vi "linear interp iiii- complex - z-omega - tails.vi"(0 "z":cdb[](array[numeric]), 5 "omega":dbl[](array[numeric]), 11 "center":i32=-1) -> (2 "directed sigma":cdb, 3 "directed sigma - abs":dbl, 4 "z out":cdb[](array[numeric]), 6 "omega out":dbl[](array[numeric]), 8 "left":cdb, 10 "center":cdb, 12 "intercept":cdb, 13 "slope":cdb, 15 "right":cdb)   [LabVIEW 2010]
uses:
  Q - not nan -- real.vi
  Q - not nan -- integer.vi
  <vilib>/Analysis/Matrix/Numeric/Conversions/Array To Matrix - RA2.vi
  <vilib>/Analysis/baseanly.llb/Real Inverse Matrix.vi
  <vilib>/Analysis/7linalg.llb/Real Eigenvalues and Vectors.vi
  <vilib>/Analysis/Matrix/Numeric/Conversions/Matrix To Array - CM.vi
  <vilib>/Analysis/baseanly.llb/Complex A x B.vi
  <vilib>/Analysis/NI_AALBase.lvlib
  <vilib>/Analysis/Matrix/NI_Matrix.lvlib
  <vilib>/Analysis/NI_AALPro.lvlib
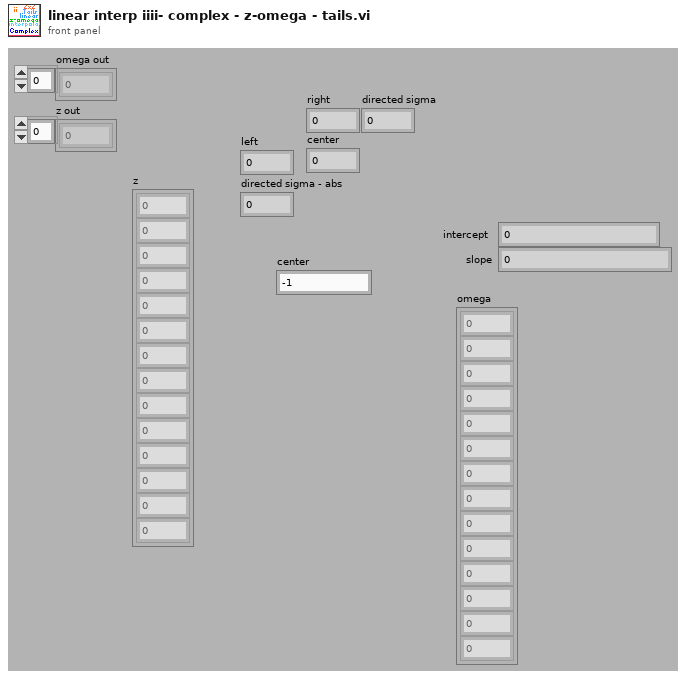
[diagram p1: front panel]
types:
  T1 = typedef "NI_Matrix.lvlib/RealMatrix.ctl" = dbl[][]
  T2 = typedef "NI_Matrix.lvlib/ComplexMatrix.ctl" = cdb[][]
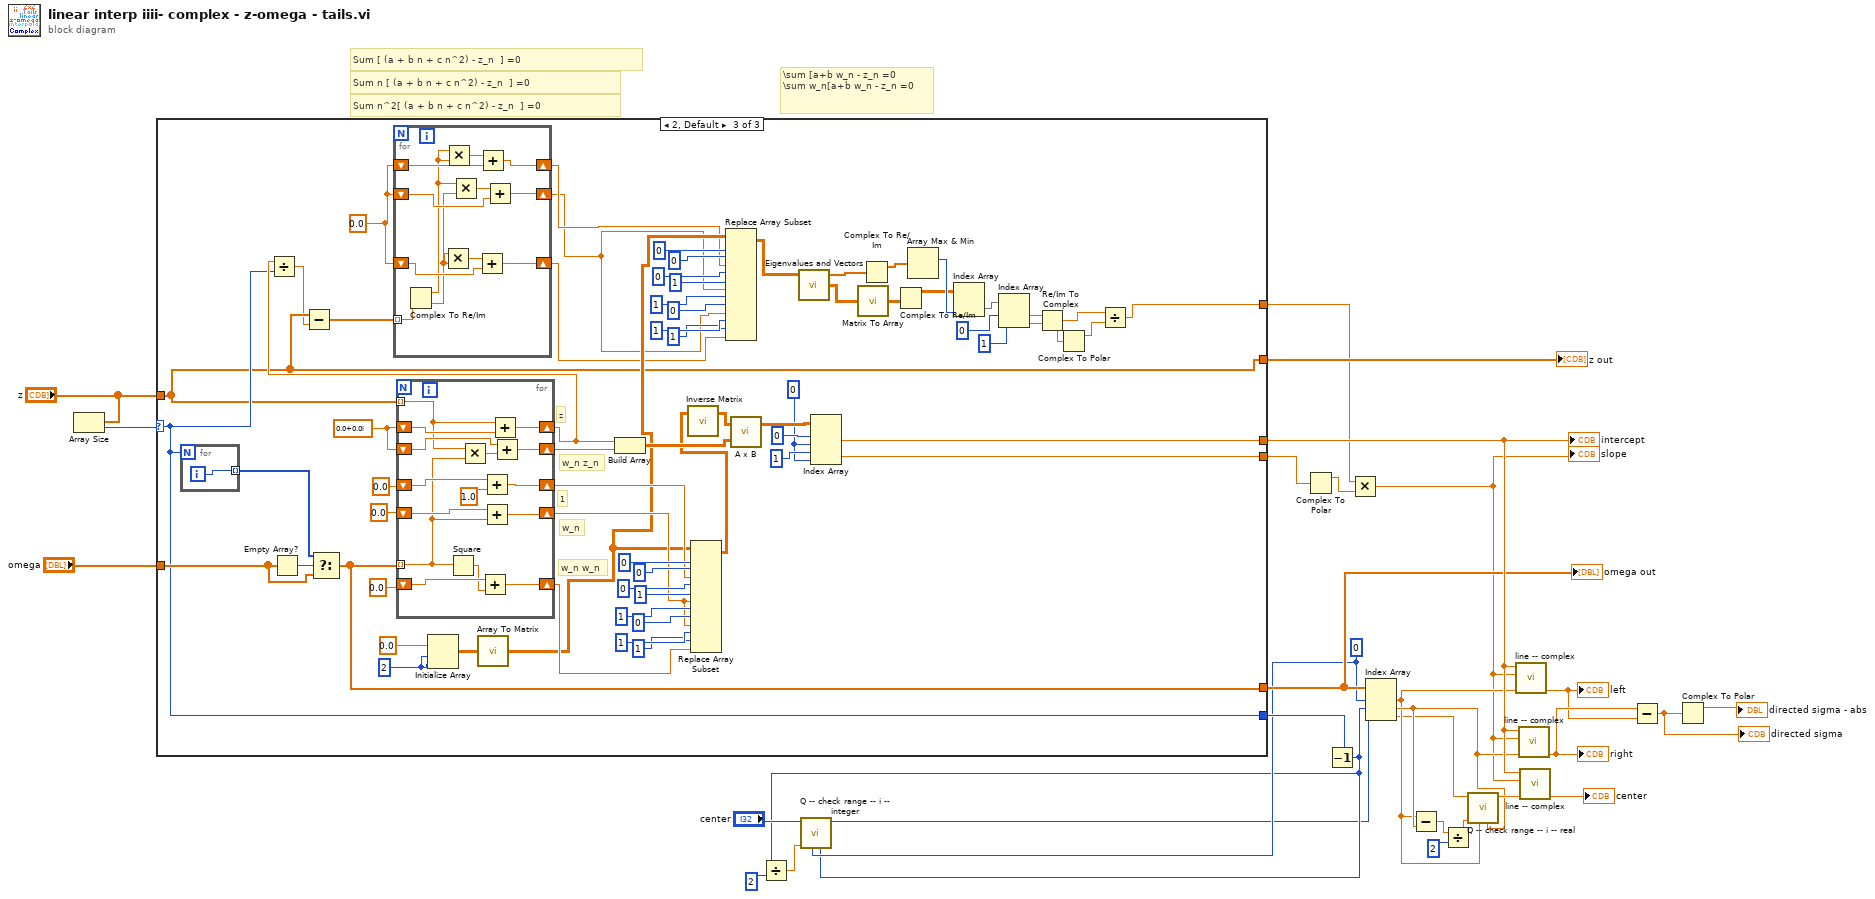
[diagram p0: block diagram]
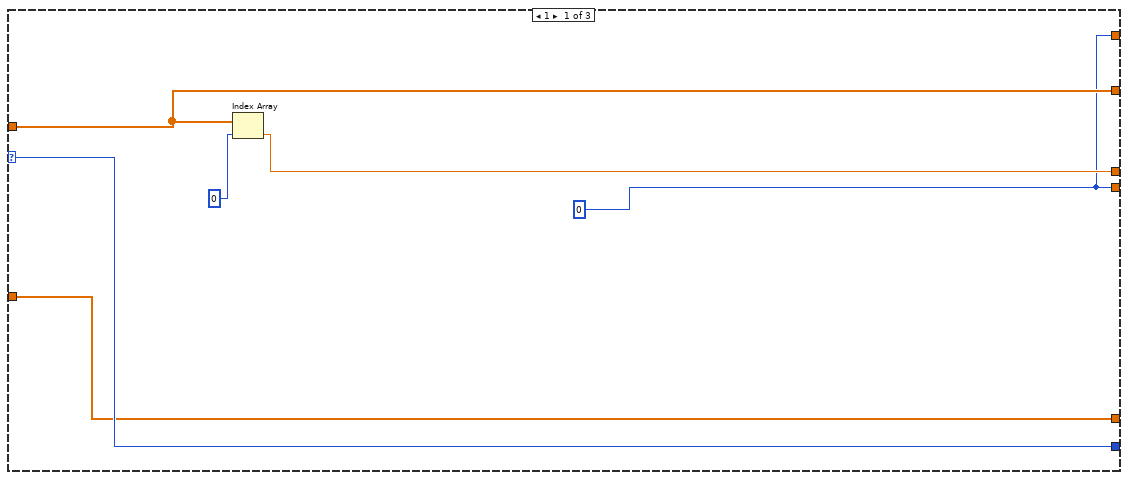
[diagram p2: hidden frame]
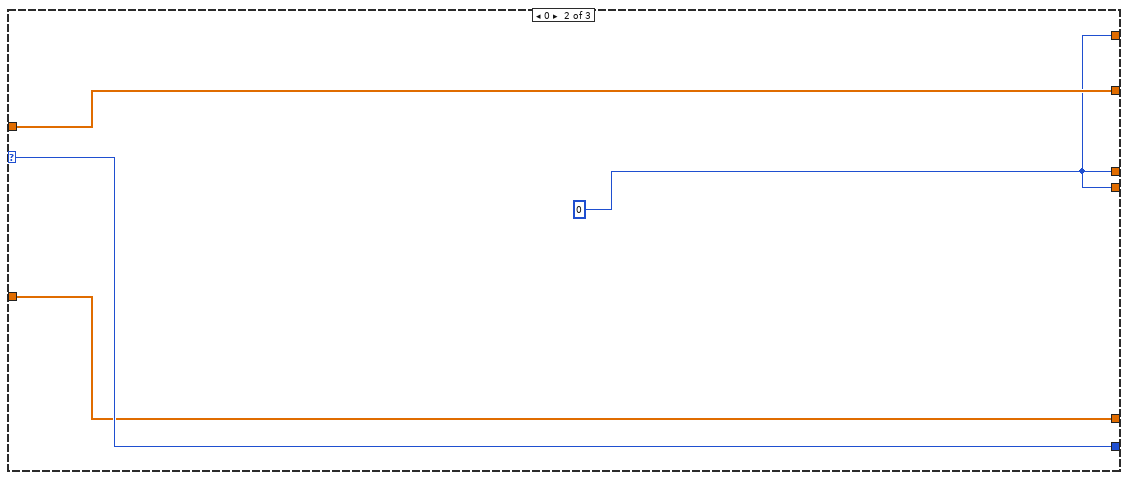
[diagram p3: hidden frame]
diagram:
  w7 = 0 ("n")
  # "\\sum [a+b w_n - z_n =0 \n\\sum w_n[a+b w_n - z_n =0"
  # "Sum n^2[ (a + b n + c n^2) - z_n  ] =0"
  # "Sum n [ (a + b n + c n^2) - z_n  ] =0"
  # "Sum [ (a + b n + c n^2) - z_n  ] =0"
  n1 = Array Size(array="z") -> (size(s)=w18:i32)
  n2 = case shown="2, Default" w18 {
    selector: w18 -> [w33 w39 w47]
    tunnel: [w34 w36 w96] -> w20
    tunnel: [w30 w36 w95] -> w4
    tunnel: "z" -> [w31 w38 w46]
    tunnel: [w33 w39 w47] -> w23
    tunnel: "omega" -> [w32 w37 w93]
    tunnel: [w32 w37 w73] -> w16
    tunnel: [w31 w38 w46] -> w15
    tunnel: [w30 w36 w40] -> w2
    frame 1 {
      w30 = 0 ("index")
      n3 = Index Array(array=w31, index=0) -> (element=w34:cdb)
    }
    frame 0 {
      w36 = 0 ("index")
    }
    frame 2, Default {
      w49 = 0.0
      w91 = 2 ("n")
      w97 = 0 ("index (row)")
      w103 = cdb 0.0+0.0i
      # "w_n w_n"
      # "w_n"
      # "1"
      # "w_n z_n"
      # "z"
      n4 = for {
        N: w47 -> [_]
        tunnel: [w117] -> w92 mode=indexing
        i -> [w117]
      }
      n5 = Empty Array?(array=w93) -> (empty?=w94:bool)
      n6 = Select(t=w92, s=w94, f=w93) -> (s? t:f=w73:dbl[])
      n7 = for {
        tunnel: w46 -> [w118] mode=indexing
        shift-right: [w132] -> w48
        shift-left: w103 -> [w131]
        shift-right: [w129] -> w102
        shift-left: w103 -> [w128]
        shift-right: [w126] -> w82
        shift-left: 0.0 -> [w127]
        shift-right: [w123] -> w77
        shift-left: 0.0 -> [w124]
        tunnel: w73 -> [w120] mode=indexing
        shift-right: [w121] -> w76
        shift-left: 0.0 -> [w122]
        n8 = Square(x=w120) -> (x^2=w119:dbl)
        n9 = Multiply(x=w118, y=w120) -> (x*y=w130:cdb)
        n10 = Add(x=w122, y=w119) -> (x+y=w121:dbl)
        n11 = Add(x=w127, y=1.0) -> (x+y=w126:dbl)
        n12 = Add(x=w124, y=w120) -> (x+y=w123:dbl)
        n13 = Add(x=w118, y=w131) -> (x+y=w132:cdb)
        n14 = Add(x=w128, y=w130) -> (x+y=w129:cdb)
      }
      n15 = Divide(x=w48, y=w47) -> (x/y=w45:cdb)
      n16 = Subtract(x=w46, y=w45) -> (x-y=w44:cdb[])
      n17 = for {
        tunnel: w44 -> [w116] mode=indexing
        shift-right: [w113] -> w43
        shift-left: w49 -> [w115]
        shift-right: [w111] -> w41
        shift-left: w49 -> [w110]
        shift-right: [w109] -> w42
        shift-left: w49 -> [w108]
        n18 = Complex To Re/Im(x + iy=w116) -> (x=w106:dbl, y=w105:dbl)
        n19 = Multiply(x=w105, y=w105) -> (x*y=w112:dbl)
        n20 = Multiply(x=w106, y=w106) -> (x*y=w114:dbl)
        n21 = Multiply(x=w106, y=w105) -> (x*y=w107:dbl)
        n22 = Add(x=w112, y=w110) -> (x+y=w111:dbl)
        n23 = Add(x=w114, y=w115) -> (x+y=w113:dbl)
        n24 = Add(x=w107, y=w108) -> (x+y=w109:dbl)
      }
      n25 = Initialize Array(0.0 ("n"), w91, w91) -> (w86:dbl[][])
      n26 = call-poly <vilib>:"Array To Matrix.vi"("Real 2D Array"=w86) -> ("Real Matrix"=w64:T1)
      n27 = Build Array(w48, w102) -> (w101:T2)
      n28 = Replace Array Subset(array=w64, new element #1=w82, index (row) #1=0 ("n"), index (col) #1=0 ("n"), new element #2=w77, index (row) #2=0 ("n"), index (col) #2=1 ("n"), new element #3=w77, index (row) #3=1 ("n"), index (col) #3=0 ("n"), new element #4=w76, index (row) #4=1 ("n"), index (col) #4=1 ("n")) -> (w75:T1)
      n29 = call-poly <vilib>:"Inverse Matrix.vi"("Input Matrix"=w75) -> ("Inverse Matrix"=w74:T1)  [unwired: 1 in, 1 out]
      n30 = Replace Array Subset(array=w64, new element #1=w43, index (row) #1=0 ("n"), index (col) #1=0 ("n"), new element #2=w42, index (row) #2=0 ("n"), index (col) #2=1 ("n"), new element #3=w42, index (row) #3=1 ("n"), index (col) #3=0 ("n"), new element #4=w41, index (row) #4=1 ("n"), index (col) #4=1 ("n")) -> (w63:T1)
      n31 = call-poly <vilib>:"A x B.vi"("B"=w101, "A"=w74) -> ("A x B"=w100:T2)  [unwired: 1 out]
      n32 = call-poly <vilib>:"Eigenvalues and Vectors.vi"("Input Matrix"=w63) -> ("Eigenvectors"=w60:T2, "Eigenvalues"=w61:cdb[])  [unwired: 2 in, 1 out]
      n33 = Index Array(array=w100, index (row) #1=0 ("index (row)"), index (col) #1=w97, index (row) #2=1 ("index (row)"), index (col) #2=w97) -> (element #1=w96:cdb, element #2=w95:cdb)
      n34 = call-poly <vilib>:"Matrix To Array.vi"("Complex Matrix"=w60) -> ("Complex 2D Array"=w62:cdb[][])
      n35 = Complex To Re/Im(x + iy=w61) -> (x=w59:dbl[])  [unwired: 1 out]
      n36 = Complex To Re/Im(x + iy=w62) -> (x=w57:dbl[][])  [unwired: 1 out]
      n37 = Array Max & Min(array=w59) -> (max index (indices)=w58:i32)  [unwired: 3 out]
      n38 = Index Array(array=w57, index (col)=w58) -> (element=w56:dbl[])  [unwired: 1 in]
      n39 = Index Array(array=w56, index #1=0 ("n"), index #2=1 ("n")) -> (element #1=w54:dbl, element #2=w55:dbl)
      n40 = Re/Im To Complex(1:w55, 2:w54) -> (0:w50:cdb)
      n41 = Complex To Polar(r * e^(i*theta)=w50) -> (r=w51:dbl)  [unwired: 1 out]
      n42 = Divide(x=w50, y=w51) -> (x/y=w40:cdb)
    }
  }
  "intercept" <- w20
  "omega out" <- w16
  "z out" <- w15
  n43 = Complex To Polar(r * e^(i*theta)=w4) -> (r=w3:dbl)  [unwired: 1 out]
  n44 = Decrement(x=w23) -> (x-1=w6:i32)
  n45 = Divide(x=w6, y=2 ("n")) -> (x/y=w9:dbl)
  n46 = call "Q -- check range -- i -- integer.vi"("upper"=w6, "lower"=w7, "default"=w9, "number"="center") -> ("number in range"=w5:i32)  [unwired: 5 in, 2 out]
  n47 = Multiply(x=w2, y=w3) -> (x*y=w1:cdb)
  "slope" <- w1
  n48 = Index Array(array=w16, index #1=w7, index #2=w6, index #3=w5) -> (element #1=w13:dbl, element #2=w14:dbl, element #3=w11:dbl)
  n49 = Subtract(x=w13, y=w14) -> (x-y=w12:dbl)
  n50 = Divide(x=w12, y=2 ("n")) -> (x/y=w24:dbl)
  n51 = call "Q -- check range -- i -- real.vi"("upper"=w14, "lower"=w13, "default"=w24, "number"=w11) -> ("number in range"=w28:dbl)  [unwired: 5 in, 2 out]
  n52 = call "line -- complex.vi"("n"=w13, "slope"=w1, "intercept"=w20) -> ("parabola"=w25:cdb)  [unwired: 7 in, 1 out]
  "left" <- w25
  n53 = call "line -- complex.vi"("n"=w14, "slope"=w1, "intercept"=w20) -> ("parabola"=w26:cdb)  [unwired: 7 in, 1 out]
  "right" <- w26
  n54 = call "line -- complex.vi"("n"=w28, "slope"=w1, "intercept"=w20) -> ("parabola"=→"center":cdb)  [unwired: 7 in, 1 out]
  n55 = Subtract(x=w26, y=w25) -> (x-y=w21:cdb)
  "directed sigma" <- w21
  n56 = Complex To Polar(r * e^(i*theta)=w21) -> (r=→"directed sigma - abs":dbl)  [unwired: 1 out]
